vi "Get Alarm Volume.vi"(8 "error IO":errorcluster, 11 "VISA resource name":refnum<visa-resource-name>) -> (0 "error Out":errorcluster, 2 "Alarm Volume":i32, 3 "VISA resource Out":refnum<visa-resource-name>)   [LabVIEW 2012, in "Associated Research 78XX Series.lvlib"]
uses:
  <instrlib>/Associated Research 78XX Series/Associated Research 78XX Series.lvlib
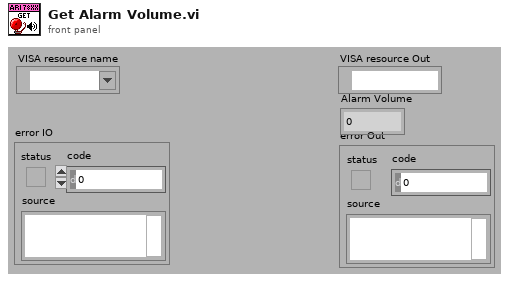
[diagram p1: front panel]
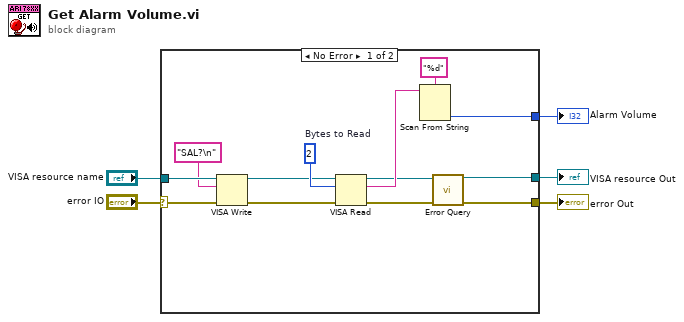
[diagram p0: block diagram]
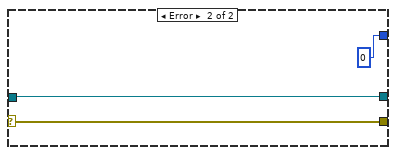
[diagram p2: hidden frame]
diagram:
  n1 = case shown="No Error" "error IO" {
    selector: "error IO" -> [w18 w21]
    tunnel: [w15 w21] -> w2
    tunnel: [w16 w20] -> w3
    tunnel: "VISA resource name" -> [w17 w20]
    tunnel: [w11 0] -> w1
    frame No Error {
      w10 = u32 2  # Bytes to Read
      n2 = VISA Write(VISA resource name=w17, write buffer="SAL?\n" ("Command to Send (empty)"), error in (no error)=w18) -> (VISA resource name out=w7:refnum<visa-resource-name>, error out=w6:errorcluster)  [unwired: 1 out]
      n3 = VISA Read(VISA resource name=w7, byte count=w10, error in (no error)=w6) -> (VISA resource name out=w9:refnum<visa-resource-name>, read buffer=w12:string, error out=w8:errorcluster)  [unwired: 1 out]
      n4 = Scan From String(format string="%d", input string=w12) -> (output 1=w11:i32)  [unwired: 3 in, 3 out]
      n5 = call <instrlib>:"Error Query.vi"("VISA resource name"=w9, "error in (no error)"=w8) -> ("VISA resource name out"=w16:refnum<visa-resource-name>, "error out"=w15:errorcluster)  [unwired: 10 in, 2 out]
    }
    frame Error {
    }
  }
  "VISA resource Out" <- w3
  "error Out" <- w2
  "Alarm Volume" <- w1
